vi "ConvertTimeStampToStrTime.vi"(10 "type":T1(ring), 11 "TimeStamp":timestamp) -> (3 "date/time string":string)   [LabVIEW 2018, in "Library-DataConvert.lvlib"]
uses:
  Library-DataConvert.lvlib
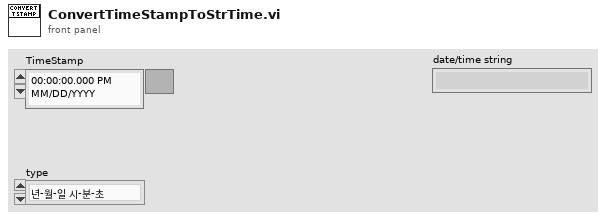
[diagram p1: front panel]
types:
  T1 = enum16{"년-월-일 시-분-초", "년-월-일", "년(2)-월(2)-일(2)", "년(2)월(2)일(2)", "년(2)-월(2)-일(2) 시-분-초", "년(4)-월(2)-일(2) 시:분:초", "년(4)-월(2)-일(2) 시:분:초.밀리초", "시(2)분(2)초(2)"}
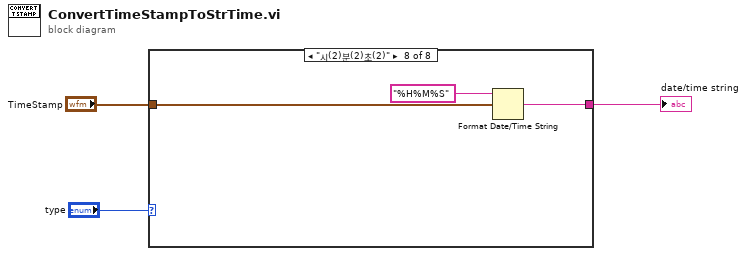
[diagram p0: block diagram]
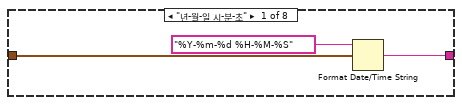
[diagram p2: hidden frame]
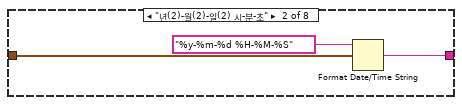
[diagram p3: hidden frame]
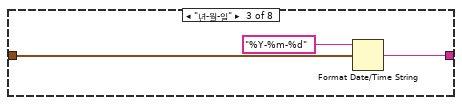
[diagram p4: hidden frame]
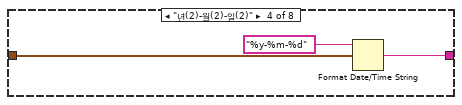
[diagram p5: hidden frame]
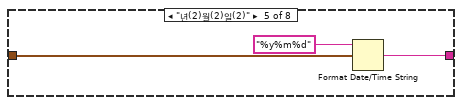
[diagram p6: hidden frame]
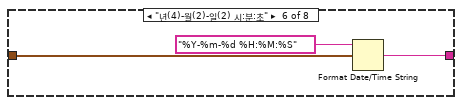
[diagram p7: hidden frame]
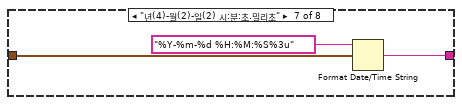
[diagram p8: hidden frame]
diagram:
  n1 = case shown="\"시(2)분(2)초(2)\"" "type" {
    tunnel: "TimeStamp" -> [w5 w8 w11 w14 w17 w20 w23 w26]
    tunnel: [w4 w7 w10 w13 w16 w19 w22 w25] -> w1
    frame "년-월-일 시-분-초" {
      n2 = Format Date/Time String(time format string (%c)="%Y-%m-%d %H-%M-%S" ("시간 포맷 문자열 (%c)"), seconds (now)=w5) -> (date/time string=w4:string)  [unwired: 1 in]
    }
    frame "년(2)-월(2)-일(2) 시-분-초" {
      n3 = Format Date/Time String(time format string (%c)="%y-%m-%d %H-%M-%S" ("시간 포맷 문자열 (%c)"), seconds (now)=w8) -> (date/time string=w7:string)  [unwired: 1 in]
    }
    frame "년-월-일" {
      n4 = Format Date/Time String(time format string (%c)="%Y-%m-%d" ("시간 포맷 문자열 (%c)"), seconds (now)=w11) -> (date/time string=w10:string)  [unwired: 1 in]
    }
    frame "년(2)-월(2)-일(2)" {
      n5 = Format Date/Time String(time format string (%c)="%y-%m-%d" ("시간 포맷 문자열 (%c)"), seconds (now)=w14) -> (date/time string=w13:string)  [unwired: 1 in]
    }
    frame "년(2)월(2)일(2)" {
      n6 = Format Date/Time String(time format string (%c)="%y%m%d" ("시간 포맷 문자열 (%c)"), seconds (now)=w17) -> (date/time string=w16:string)  [unwired: 1 in]
    }
    frame "년(4)-월(2)-일(2) 시:분:초" {
      n7 = Format Date/Time String(time format string (%c)="%Y-%m-%d %H:%M:%S" ("시간 포맷 문자열 (%c)"), seconds (now)=w20) -> (date/time string=w19:string)  [unwired: 1 in]
    }
    frame "년(4)-월(2)-일(2) 시:분:초.밀리초" {
      n8 = Format Date/Time String(time format string (%c)="%Y-%m-%d %H:%M:%S%3u" ("시간 포맷 문자열 (%c)"), seconds (now)=w23) -> (date/time string=w22:string)  [unwired: 1 in]
    }
    frame "시(2)분(2)초(2)" {
      n9 = Format Date/Time String(time format string (%c)="%H%M%S" ("시간 포맷 문자열 (%c)"), seconds (now)=w26) -> (date/time string=w25:string)  [unwired: 1 in]
    }
  }
  "date/time string" <- w1
